vi "Prompt FG.vi"(7 "ExecAnchor":refnum<class "ExecAnchor.lvclass">, 10 "Clear":bool, 11 "Set":bool) -> (3 "Acquired":bool)   [LabVIEW 2020, in "VolatusGUI.lvlib" / "GUI Element.lvclass"]
uses:
  GUI Element.lvclass
  lv-exec-anchor/ExecAnchor/ExecAnchor.lvclass
  lv-exec-anchor/ExecAnchor/ExecAnchor.lvclass/ExecAnchor.ctl
  GUI Element.lvclass/GUI Element.ctl
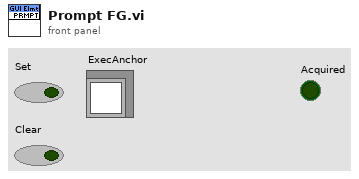
[diagram p1: front panel]
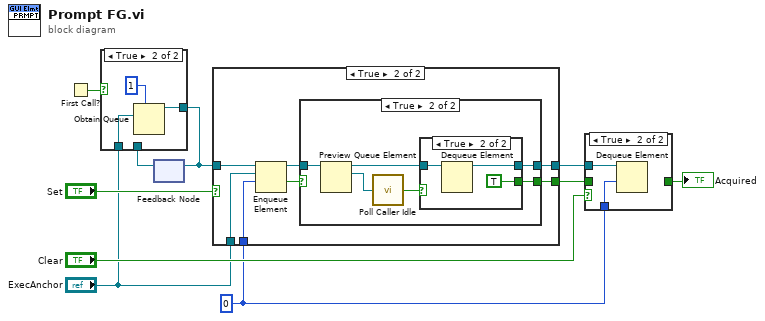
[diagram p0: block diagram]
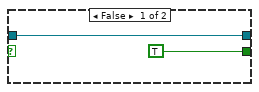
[diagram p4: hidden frame]
diagram:
  w4 = 0 ("timeout in ms (-1)")
  n1 = First Call?() -> (First Call?: T/F=w10:bool)
  n2 = feedback #1() -> (w9:refnum<queue>)  [unwired: 1 in]
  n3 = case shown="True" w10 {
    tunnel: [w11 w13] -> w7
    tunnel: w9 -> [w11 _]
    tunnel: "ExecAnchor" -> [_ w12]
    frame False {
    }
    frame True {
      n4 = Obtain Queue(max queue size (-1, unlimited)=1, element data type=w12) -> (queue out=w13:refnum<queue>)  [unwired: 3 in, 2 out]
    }
  }
  n5 = feedback-in #1(w7) -> ()
  n6 = case shown="True" "Set" {
    tunnel: w7 -> [w15 w22]
    tunnel: [_ w16] -> w3
    tunnel: [w15 w17] -> w5
    tunnel: w4 -> [_ w21]
    tunnel: "ExecAnchor" -> [_ w20]
    frame False {
    }
    frame True {
      n7 = Enqueue Element(queue=w22, element=w20, timeout in ms (-1)=w21) -> (queue out=w18:refnum<queue>, timed out?=w19:bool)  [unwired: 1 in, 1 out]
      n8 = case shown="True" w19 {
        tunnel: w18 -> [w24 w30]
        tunnel: [w24 w28] -> w17
        tunnel: [TRUE w27] -> w16
        frame False {
        }
        frame True {
          n9 = Preview Queue Element(queue=w30) -> (queue out=w29:refnum<queue>, element=w26:refnum<class "ExecAnchor.lvclass">)  [unwired: 2 in, 2 out]
          n10 = call "Poll Caller Idle.vi"("ExecAnchor in"=w26) -> ("Caller Idle"=w25:bool)  [unwired: 3 in, 1 out]
          n11 = case shown="True" w25 {
            tunnel: w29 -> [w31 w34]
            tunnel: [w31 w33] -> w28
            tunnel: [_ TRUE] -> w27
            frame False {
            }
            frame True {
              n12 = Dequeue Element(queue=w34) -> (queue out=w33:refnum<queue>)  [unwired: 2 in, 3 out]
            }
          }
        }
      }
    }
  }
  n13 = case shown="True" "Clear" {
    tunnel: w5 -> [_ w37]
    tunnel: w4 -> [_ w36]
    tunnel: w3 -> [w35 _]
    tunnel: [w35 _] -> w2
    frame False {
    }
    frame True {
      n14 = Dequeue Element(queue=w37, timeout in ms (-1)=w36) -> ()  [unwired: 1 in, 4 out]
    }
  }
  "Acquired" <- w2
